vi "Position.vi"   [LabVIEW 2013]
uses:
  Robot Global Data.vi
types:
  T1 = typedef "Semaphore RefNum" = refnum<k1>
  T2 = typedef "WPI_GyroDevRef.ctl" = cluster{"DevStatus":errorcluster, "Analog Module":T3, "Analog Channel":T4, "Offset":dbl, "Gain (VoltsPerDegree/Second)":dbl}
  T3 = typedef "FPGA_TypedefAnalogModule.ctl" = enum16{"Analog Module 1", "Analog Module 2"}
  T4 = typedef "FPGA_AIChannel.ctl" = enum8{"AI 1", "AI 2", "AI 3", "AI 4", "AI 5", "AI 6", "AI 7", "AI 8", "Invalid"}
  T5 = typedef "WPI_EncoderDevRef.ctl" = cluster{"DevStatus":errorcluster, "EncoderIndex":T6, "CounterIndex":T7, "DistancePerCount":dbl, "Decoding Type":T8}
  T6 = typedef "FPGA_EncoderIdx.ctl" = enum8{"Enc 0", "Enc 1", "Enc 2", "Enc 3", "Invalid"}
  T7 = typedef "FPGA_CounterCtrSystemIndex.ctl" = enum8{"Ctr 0", "Ctr 1", "Ctr 2", "Ctr 3", "Ctr 4", "Ctr 5", "Ctr 6", "Ctr 7", "Invalid"}
  T8 = typedef "WPI_EncoderType.ctl" = enum16{"1x", "2x", "4x"}
  T9 = typedef "Position Typedef.ctl" = cluster{"X":dbl, "Y":dbl, "Heading":dbl}
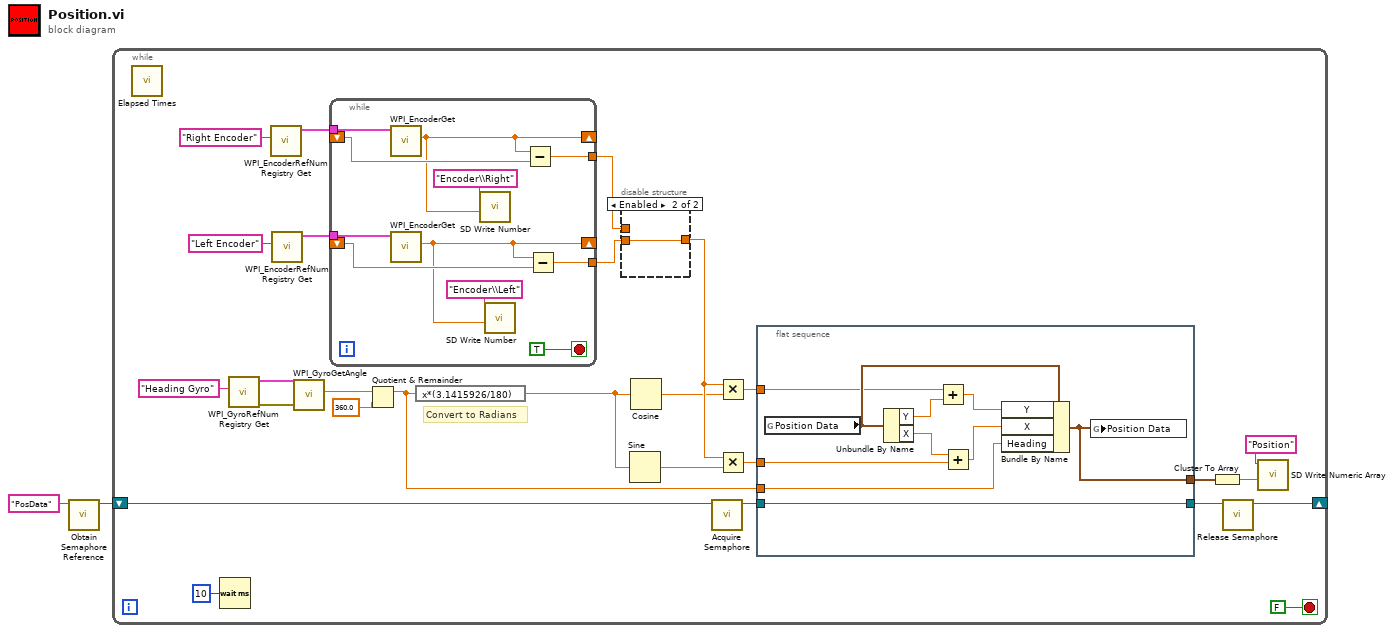
[diagram p0: block diagram]
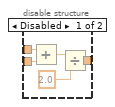
[diagram p2: hidden frame]
diagram:
  n1 = call <vilib>:"Obtain Semaphore Reference.vi"("name (unnamed)"="PosData") -> ("semaphore"=w1:T1)  [unwired: 4 in, 2 out]
  n2 = while {
    shift-right: [w6] -> _
    shift-left: w1 -> [w4]
    stop <- FALSE stop-if-true
    # "Convert to Radians"
    n3 = call "Elapsed Times.vi"() -> ()  [unwired: 3 in, 1 out]
    n4 = Wait (ms)(milliseconds to wait=u32 10) -> ()  [unwired: 1 out]
    n5 = call <vilib>:"WPI_GyroRefNum Registry Get.vi"("refnum name"="Heading Gyro") -> ("error out"=w23:errorcluster, "GyroDevRef"=w22:T2)  [unwired: 1 in, 8 out]
    n6 = call <vilib>:"WPI_EncoderRefNum Registry Get.vi"("refnum name"="Right Encoder") -> ("EncoderDevRef"=w15:T5)  [unwired: 1 in, 9 out]
    n7 = call <vilib>:"WPI_EncoderRefNum Registry Get.vi"("refnum name"="Left Encoder") -> ("EncoderDevRef"=w16:T5)  [unwired: 1 in, 9 out]
    n8 = call <vilib>:"WPI_GyroGetAngle.vi"("error in (no error)"=w23, "GyroDevRef"=w22) -> ("Angle"=w19:dbl)  [unwired: 9 out]
    n9 = while {
      tunnel: w15 -> [w56]
      tunnel: w16 -> [w55]
      shift-right: [w48] -> _
      shift-left: _ -> [w54]
      shift-right: [w46] -> _
      shift-left: _ -> [w53]
      tunnel: [w52] -> w17
      tunnel: [w51] -> w18
      stop <- TRUE stop-if-true
      n10 = call <vilib>:"WPI_EncoderGet.vi"("EncoderDevRef"=w56) -> ("Distance"=w48:dbl)  [unwired: 1 in, 9 out]
      n11 = call <vilib>:"WPI_EncoderGet.vi"("EncoderDevRef"=w55) -> ("Distance"=w46:dbl)  [unwired: 1 in, 9 out]
      n12 = call <vilib>:"SD Write Number.vi"("Numeric"=w48, "Name"="Encoder\\Right") -> ()  [unwired: 8 in, 2 out]
      n13 = call <vilib>:"SD Write Number.vi"("Numeric"=w46, "Name"="Encoder\\Left") -> ()  [unwired: 8 in, 2 out]
      n14 = Subtract(x=w48, y=w54) -> (x-y=w52:dbl)
      n15 = Subtract(x=w46, y=w53) -> (x-y=w51:dbl)
    }
    n16 = Quotient & Remainder(x=w19, y=360.0) -> (x-y*floor(x/y)=w29:dbl)  [unwired: 1 out]
    n17 = expression code="x*(3.1415926/180)"(w29) -> (w21:dbl)
    n18 = disable-structure shown="Enabled" {
      disable-tunnel: [w44 w45] -> w25
      disable-tunnel: w18 -> [w43 w45]
      disable-tunnel: w17 -> [w42 _]
      frame Disabled {
        n19 = Add(x=w42, y=w43) -> (x+y=w40:dbl)
        n20 = Divide(x=w40, y=2.0) -> (x/y=w44:dbl)
      }
      frame Enabled {
      }
    }
    n21 = Sine(x=w21) -> (sin(x)=w26:dbl)
    n22 = Cosine(x=w21) -> (cos(x)=w24:dbl)
    n23 = call <vilib>:"Acquire Semaphore.vi"("semaphore"=w4) -> ("semaphore out"=w11:T1)  [unwired: 4 in, 2 out]
    n24 = Multiply(x=w25, y=w24) -> (x*y=w27:dbl)
    n25 = Multiply(x=w25, y=w26) -> (x*y=w28:dbl)
    n26 = flat-sequence {
      tunnel: w29 -> [w39]
      tunnel: w28 -> [w34]
      tunnel: w27 -> [w32]
      tunnel: w11 -> [w30]
      tunnel: [w31] -> w9
      tunnel: [w30] -> w8
      frame #0 {
        n27 = global read "Robot Global Data.vi" "Position Data"() -> (w36:T9)
        n28 = Unbundle By Name(w36) -> ("Y"=w33:dbl, "X"=w35:dbl)
        n29 = Add(x=w32, y=w33) -> (x+y=w37:dbl)
        n30 = Add(x=w35, y=w34) -> (x+y=w38:dbl)
        n31 = Bundle By Name(cluster=w36, "Y"=w37, "X"=w38, "Heading"=w39) -> (w31:T9)
        n32 = global write "Robot Global Data.vi" "Position Data"(w31) -> ()
      }
    }
    n33 = Cluster To Array(cluster=w9) -> (array=w10:dbl[])
    n34 = call <vilib>:"Release Semaphore.vi"("semaphore"=w8) -> ("semaphore out"=w6:T1)  [unwired: 5 in, 1 out]
    n35 = call <vilib>:"SD Write Numeric Array.vi"("Numeric Array"=w10, "Name"="Position") -> ()  [unwired: 8 in, 2 out]
  }
